vi "GetSetAutoArray.vi"(9 "Array":string[](array[string]), 10 "String":string, 11 "Mode":enum16{"Get", "Add String", "Add String Array"}(ring)) -> (3 "Auto List":string[](array[string]))   [LabVIEW 2016, in "BB_AutonomousSelector.lvlib"]
uses:
  BB_AutonomousSelector.lvlib
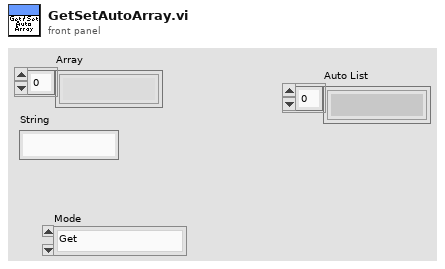
[diagram p1: front panel]
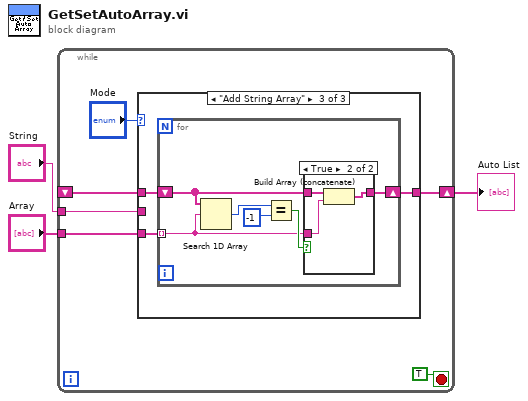
[diagram p0: block diagram]
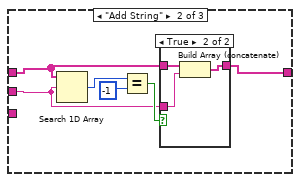
[diagram p3: hidden frame]
diagram:
  n1 = while {
    shift-right: [w6] -> w3
    shift-left: _ -> [w7]
    tunnel: "String" -> [w5]
    tunnel: "Array" -> [w4]
    stop <- TRUE stop-if-true
    n2 = case shown="\"Add String Array\"" "Mode" {
      tunnel: w7 -> [w10 w13 w23]
      tunnel: [w10 w11 w21] -> w6
      tunnel: w5 -> [_ w12 _]
      tunnel: w4 -> [_ _ w22]
      frame "Get", Default {
      }
      frame "Add String" {
        n3 = Search 1D Array(1D array=w13, element=w12) -> (index of element=w16:i32)  [unwired: 1 in]
        n4 = Equal?(x=w16, y=-1) -> (x = y?=w14:bool)
        n5 = case shown="True" w14 {
          tunnel: w13 -> [w17 w20]
          tunnel: [w17 w18] -> w11
          tunnel: w12 -> [_ w19]
          frame False {
          }
          frame True {
            n6 = Build Array (concatenate)(w20, w19) -> (w18:string[])
          }
        }
      }
      frame "Add String Array" {
        n7 = for {
          tunnel: w22 -> [w25] mode=indexing
          shift-right: [w24] -> w21
          shift-left: w23 -> [w29]
          n8 = Search 1D Array(1D array=w29, element=w25) -> (index of element=w28:i32)  [unwired: 1 in]
          n9 = Equal?(x=w28, y=-1) -> (x = y?=w26:bool)
          n10 = case shown="True" w26 {
            tunnel: w29 -> [w30 w33]
            tunnel: [w30 w31] -> w24
            tunnel: w25 -> [_ w32]
            frame False {
            }
            frame True {
              n11 = Build Array (concatenate)(w33, w32) -> (w31:string[])
            }
          }
        }
      }
    }
  }
  "Auto List" <- w3
